vi "GetAllComicsBySeries.vi"(6 "Run as sub":bool, 8 "error in (no error)":errorcluster, 11 "timeout (0 = Use Default)":i32=60000) -> (0 "error IO":errorcluster)   [LabVIEW 2024]
panel:
  out "current folder":string
  out "retries":i32
  in  "Folder Path":path=path "D:/Comics/Marvel"
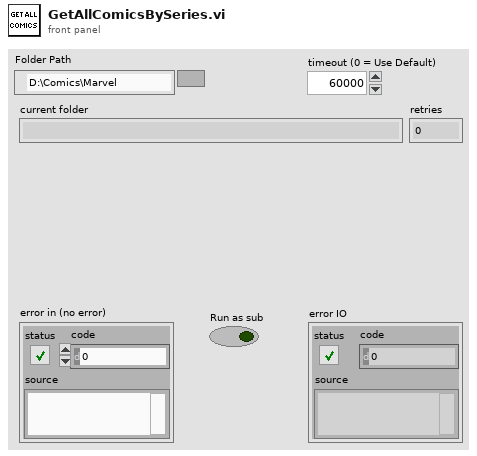
[diagram p1: front panel]
types:
  T1 = enum32{"Invalid", "Standard", "Closed", "Hidden", "Minimized", "Maximized"}
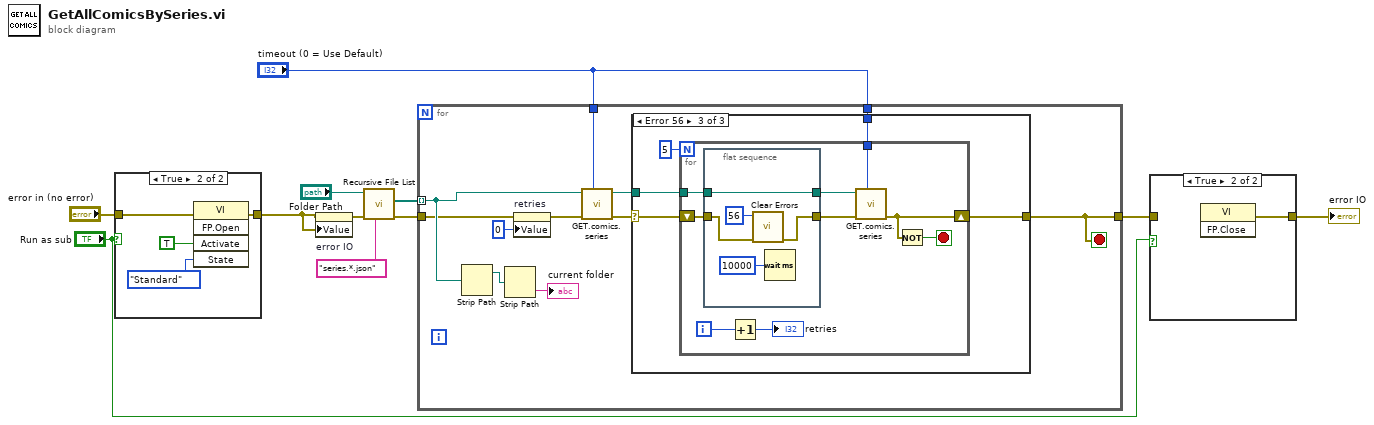
[diagram p0: block diagram]
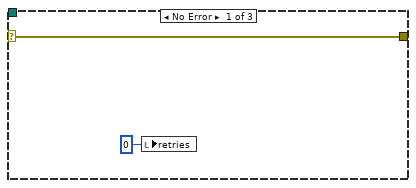
[diagram p4: hidden frame]
diagram:
  n1 = case shown="True" "Run as sub" {
    tunnel: "error in (no error)" -> [w12 w14]
    tunnel: [w12 w13] -> w4
    frame False {
    }
    frame True {
      n2 = invoke class="VI" method="FP.Open"(error in=w14, "Activate"=TRUE ("Activate?"), "State"=T1."Standard") -> (error out=w13:errorcluster)  [unwired: 2 in, 4 out]
    }
  }
  n3 = property on="error IO" class="Clust (strict)"(error in=w4, "Value"=w4) -> (error out=w7:errorcluster)  [unwired: 1 in, 1 out]
  n4 = call <vilib>:"Recursive File List.vi"("pattern"="series.*.json", "error in (no error)"=w7, "Folder Path"="Folder Path") -> ("error out"=w9:errorcluster, "All Files in Dir"=w8:path[])  [unwired: 4 in, 3 out]
  n5 = for {
    tunnel: w9 -> [w21]
    tunnel: w8 -> [w24] mode=indexing
    tunnel: [w26] -> w3
    tunnel: "timeout (0 = Use Default)" -> [w18]
    tunnel: "timeout (0 = Use Default)" -> [w17]
    stop <- w26 stop-if-true
    n6 = Strip Path(path=w24) -> (stripped path=w23:path)  [unwired: 1 out]
    n7 = Strip Path(path=w23) -> (name=→"current folder":string)  [unwired: 1 out]
    n8 = property on="retries" class="DigNum (strict)"(error in=w21, "Value"=0 ("retries")) -> (error out=w20:errorcluster)  [unwired: 1 in, 1 out]
    n9 = call "GET.comics.series.vi"("timeout (0 = Use Default)"=w18, "error in (no error)"=w20, "series json path"=w24) -> ("error out"=w27:errorcluster, "series json path 2"=w25:path)  [unwired: 7 in]
    n10 = case shown="Error 56" w27 {
      selector: w27 -> [w29 w30 w34]
      tunnel: [w29 w30 w32] -> w26
      tunnel: w25 -> [_ _ w33]
      tunnel: w17 -> [_ _ w31]
      frame No Error {
        n11 = local write "retries"(0 ("retries")) -> ()
      }
      frame Default {
      }
      frame Error {
        n12 = for {
          N: 5 -> [_]
          shift-right: [w40] -> w32
          shift-left: w34 -> [w44]
          tunnel: w33 -> [w43]
          tunnel: w31 -> [w36]
          i -> [w38]
          stop <- w39 stop-if-true
          n13 = flat-sequence {
            tunnel: w44 -> [w48]
            tunnel: [w46] -> w42
            tunnel: w43 -> [w45]
            tunnel: [w45] -> w41
            frame #0 {
              n14 = call <vilib>:"Clear Errors.vi"("error in (no error)"=w48, "specific error code to clear (0: all)"=56) -> ("error out"=w46:errorcluster)  [unwired: 4 in, 1 out]
              n15 = Wait (ms)(milliseconds to wait=u32 10000) -> ()  [unwired: 1 out]
            }
          }
          n16 = Increment(x=w38) -> (x+1=→"retries":i32)
          n17 = call "GET.comics.series.vi"("timeout (0 = Use Default)"=w36, "error in (no error)"=w42, "series json path"=w41) -> ("error out"=w40:errorcluster)  [unwired: 7 in, 1 out]
          n18 = Not(x=w40) -> (.not. x?=w39:bool)
        }
      }
    }
  }
  n19 = case shown="True" "Run as sub" {
    tunnel: w3 -> [w50 _]
    tunnel: [w50 w51] -> w1
    frame False {
    }
    frame True {
      n20 = invoke class="VI" method="FP.Close"() -> (error out=w51:errorcluster)  [unwired: 3 in, 2 out]
    }
  }
  "error IO" <- w1
